vi "ADIS16448 Loop.vi"(8 "error in":errorcluster) -> ()   [LabVIEW 2019]
uses:
  Typedef/ADIS16448 Device Reference.ctl
  Typedef/ADIS16448 Hardware Configuration.ctl
  <vilib>/Rock Robotics/WPI/SPI/WPI_SPIMode.ctl
  <vilib>/Rock Robotics/SystemInterfaces/DIO/FPGA_DIOChannel.ctl
  <vilib>/Rock Robotics/SystemInterfaces/spilib/spi_bus.ctl
  Typedef/ADIS16448 Status.ctl
  Typedef/ADIS16448 Data.ctl
  Typedef/ADIS16448 Process.ctl
  Typedef/ADIS16448 Command Type.ctl
  <vilib>/Rock Robotics/SystemInterfaces/CounterEncoderSourceConvertion/FPGA_CounterEncoderSourceConvertionLVSourceType.ctl
  <vilib>/Rock Robotics/SystemInterfaces/DIO/FPGA_DIODigitalSourceChannel.ctl
  <vilib>/Rock Robotics/SystemInterfaces/AnalogTrigger/FPGA_AnalogTriggerIndex.ctl
  <vilib>/Rock Robotics/SystemInterfaces/AnalogTrigger/FPGA_AnalogTriggerOutType.ctl
  <vilib>/Rock Robotics/WPI/SPI/WPI_SPIDevRef.ctl
  Typedef/ADIS16448 Register.ctl
  <vilib>/Rock Robotics/WPI/Counter/WPI_CounterDigitalInputToDigitalSource.vi
  <vilib>/ptbypt/NI_PtbyPt.lvlib
panel:
  in  "Calibration Time":i32
  in  "element":T1
  in  "ADIS16448DevRef":T2={"DevStatus"={"status"=FALSE, "code"=0, "source"=""}, "Hardware Config"={"SPI Clock Rate (Hz)"=1000000.0, "IMU SPI Mode (3)"=enum."Mode 3 (Clk Idle High,Sample on Trailing)", "IMU Reset Pin"=enum."SPI Port CS2", "IMU SPI Bus"=enum."SPI On-Board, CS0", "IMU Data Ready Pin"=enum."SPI Port CS1", "Stall Config"={"Pow2BytesPerRead"=255, "StallTicks"=640, "CsToSclkTicks"=5}, "IMU Status LED Pin"=enum."DIO MXP 9"}, "Calibration Complete"=refnum, "Status FIFO"=refnum, "Last Value Reference"=refnum, "Sychronous Process VI"=refnum, "Cmd FIFO"=refnum, "Source"={"DevStatus"={"status"=FALSE, "code"=0, "source"=""}, "AnalogTriggerMode?"=FALSE, "DigitalMode"={"DIO Channel"=enum."Disabled"}, "AnalogTriggerMode"={"AnalogTriggerIndex"=enum."Trig 0", "OutputType"=enum."InWindow"}}, "Data FIFO"=refnum, "IMU Status LED Pin"=enum."DIO MXP 9", "Calibration Time"=5}
  in  "Main Name":string
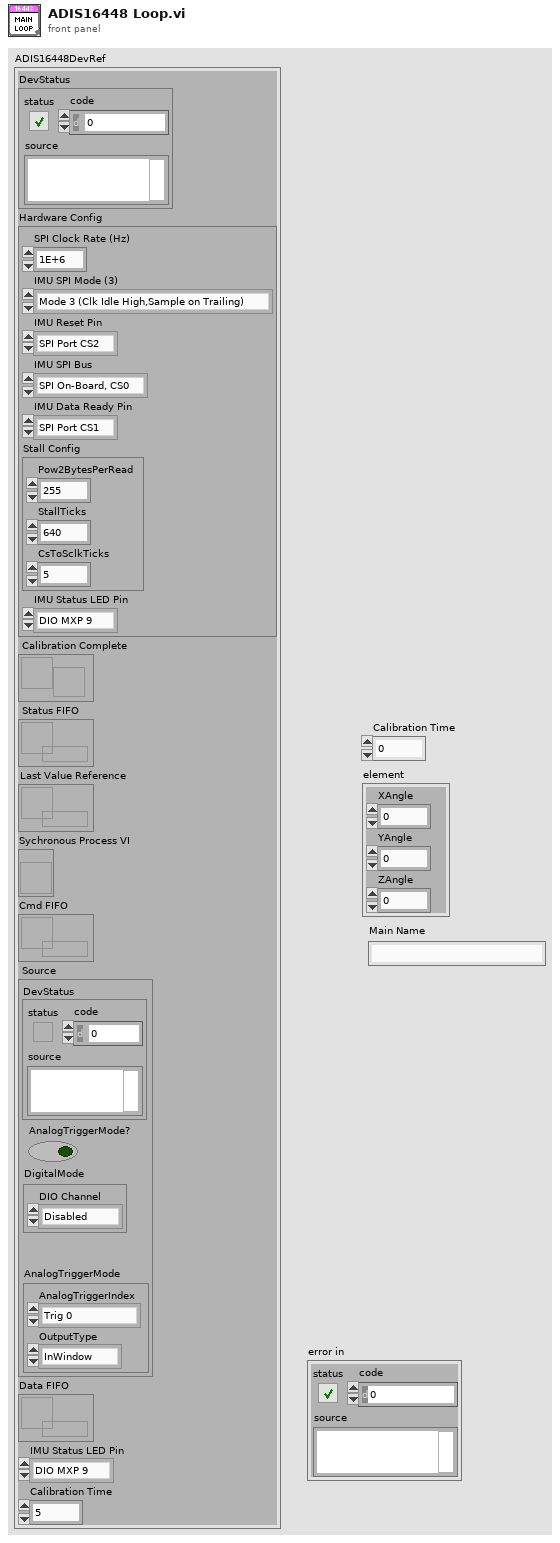
[diagram p1: front panel]
types:
  T1 = typedef "ADIS16448 Data.ctl" = cluster{"XAngle":dbl, "YAngle":dbl, "ZAngle":dbl}
  T2 = typedef "ADIS16448 Device Reference.ctl" = cluster{"DevStatus":errorcluster, "Hardware Config":T3, "Calibration Complete":refnum<notifier>, "Status FIFO":refnum<k33>, "Last Value Reference":refnum<data-value>, "Sychronous Process VI":T7, "Cmd FIFO":refnum<k33>, "Source":T8, "Data FIFO":refnum<k33>, "IMU Status LED Pin":T5, "Calibration Time":u32}
  T3 = typedef "ADIS16448 Hardware Configuration.ctl" = cluster{"SPI Clock Rate (Hz)":dbl, "IMU SPI Mode (3)":T4, "IMU Reset Pin":T5, "IMU SPI Bus":T6, "IMU Data Ready Pin":T5, "Stall Config":cluster{"Pow2BytesPerRead":u8, "StallTicks":u16, "CsToSclkTicks":u8}, "IMU Status LED Pin":T5}
  T4 = typedef "WPI_SPIMode.ctl" = enum16{"Mode 0 (Clk Idle Low,Sample on Leading)", "Mode 1 (Clk Idle Low,Sample on Trailing)", "Mode 2 (Clk Idle High,Sample on Leading)", "Mode 3 (Clk Idle High,Sample on Trailing)"}
  T5 = typedef "FPGA_DIOChannel.ctl" = enum8{"DIO 0", "DIO 1", "DIO 2", "DIO 3", "DIO 4", "DIO 5", "DIO 6", "DIO 7", "DIO 8", "DIO 9", "DIO MXP 0", "DIO MXP 1", "DIO MXP 2", "DIO MXP 3", "DIO MXP 4", "DIO MXP 5", "DIO MXP 6", "DIO MXP 7", "DIO MXP 8", "DIO MXP 9", "DIO MXP 10", "DIO MXP 11", "DIO MXP 12", "DIO MXP 13", "DIO MXP 14", "DIO MXP 15", "SPI Port CS1", "SPI Port CS2", "SPI Port CS3", "SPI Port MISO", "SPI Port MOSI", "Invalid"}
  T6 = typedef "spi_bus.ctl" = enum16{"SPI On-Board, CS0", "SPI On-Board, CS1", "SPI On-Board, CS2", "SPI On-Board, CS3", "SPI MXP", "Invalid"}
  T7 = typedef "ADIS16448 Process.ctl" = refnum<vi>
  T8 = typedef "FPGA_CounterEncoderSourceConvertionLVSourceType.ctl" = cluster{"DevStatus":errorcluster, "AnalogTriggerMode?":bool, "DigitalMode":cluster{"DIO Channel":T9}, "AnalogTriggerMode":cluster{"AnalogTriggerIndex":T10, "OutputType":T11}}
  T9 = typedef "FPGA_DIODigitalSourceChannel.ctl" = enum8{"DIO 0", "DIO 1", "DIO 2", "DIO 3", "DIO 4", "DIO 5", "DIO 6", "DIO 7", "DIO 8", "DIO 9", "DIO MXP 0", "DIO MXP 1", "DIO MXP 2", "DIO MXP 3", "DIO MXP 4", "DIO MXP 5", "DIO MXP 6", "DIO MXP 7", "DIO MXP 8", "DIO MXP 9", "DIO MXP 10", "DIO MXP 11", "DIO MXP 12", "DIO MXP 13", "DIO MXP 14", "DIO MXP 15", "SPI Port CS1", "SPI Port CS2", "SPI Port CS3", "SPI Port MISO", "SPI Port MOSI", "Disabled"}
  T10 = typedef "FPGA_AnalogTriggerIndex.ctl" = enum8{"Trig 0", "Trig 1", "Trig 2", "Trig 3", "Trig 4", "Trig 5", "Trig 6", "Trig 7", "Invalid"}
  T11 = typedef "FPGA_AnalogTriggerOutType.ctl" = enum16{"InWindow", "TriggerState", "Rising", "Falling"}
  T12 = typedef "WPI_SPIDevRef.ctl" = cluster{"DevStatus":errorcluster, "Handle":i32, "SPI Bus":T6}
  T13 = cluster{"SPIDevRef":T12, "Data Counter":u16, "Reset":bool, "Digital Source":T8, "Bytes Per Sample":u32, "Data":dbl[], "ADIS16448DevRef":T2, "TimeStampPrev":u32, "Sensor to Robot Rotation":dbl[][], "AutoSPI Active?":bool, "Offsets":dbl[], "Offset Counter":i32, "Data Header":u8[], "Zero Byte Count":u8, "Running Offset":dbl[]}
  T14 = typedef "ADIS16448 Status.ctl" = cluster{"Calibrated?":bool, "IMU Detected?":bool}
  T15 = typedef "ADIS16448 Register.ctl" = u8
  T16 = typedef "ADIS16448 Command Type.ctl" = cluster{"Command":enum16{"None", "Reset", "Rewrite Config", "Start Recal", "Recalibrate", "Recal Complete", "Exit Auto SPI", "Start Auto SPI", "Configure Cal"}, "Data":u32}
  T17 = typedef "WPI_DigitalOutputDevRef.ctl" = cluster{"DIO Channel":T5, "DevStatus":errorcluster}
  T18 = typedef "WPI_DigitalInputDevRef.ctl" = cluster{"DevStatus":errorcluster, "DIO Channel":T5}
  T19 = cluster{"Pow2BytesPerRead":u8, "StallTicks":u16, "CsToSclkTicks":u8}
  T20 = enum16{"None", "Reset", "Rewrite Config", "Start Recal", "Recalibrate", "Recal Complete", "Exit Auto SPI", "Start Auto SPI", "Configure Cal"}
  T21 = enum32{"Bad", "Idle", "Run top level", "Running"}
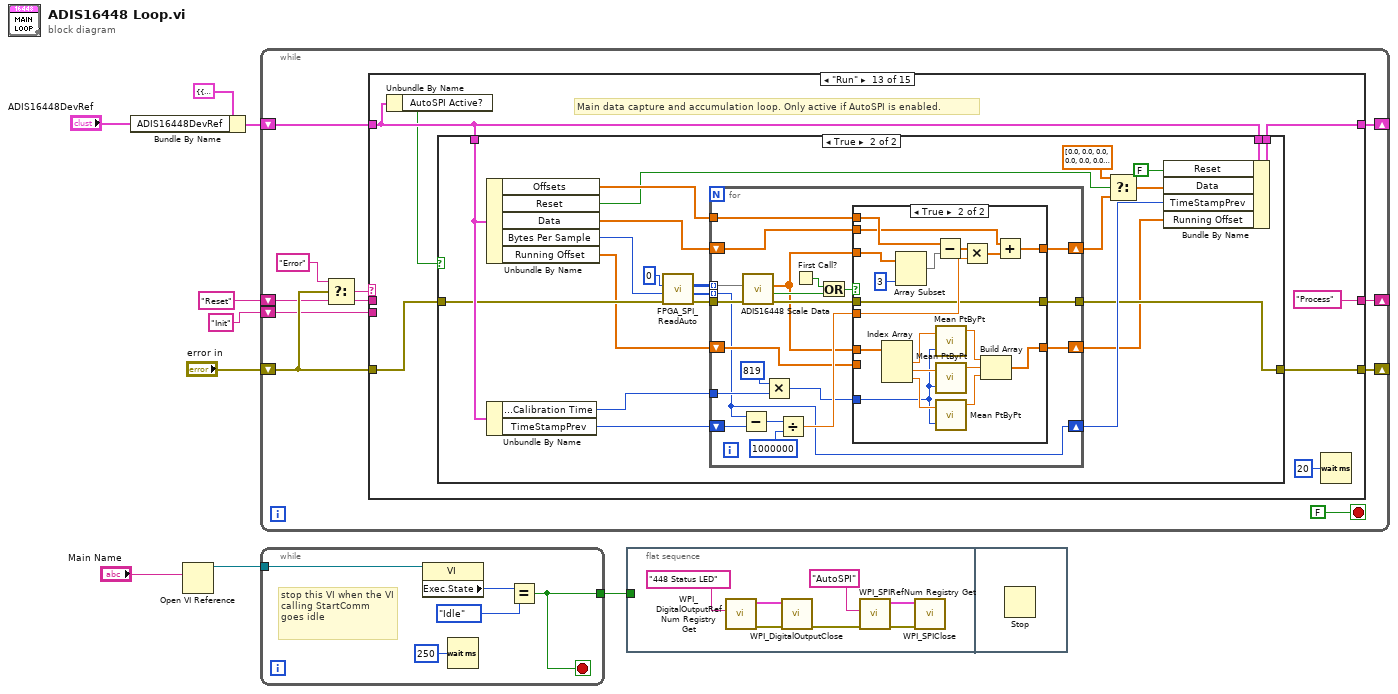
[diagram p0: block diagram]
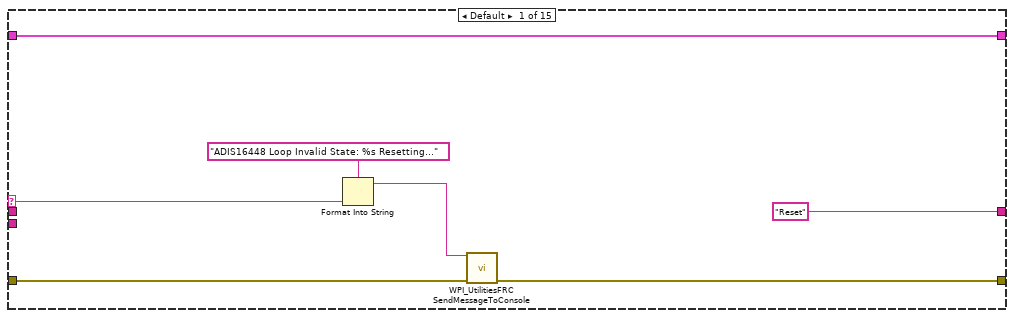
[diagram p2: hidden frame]
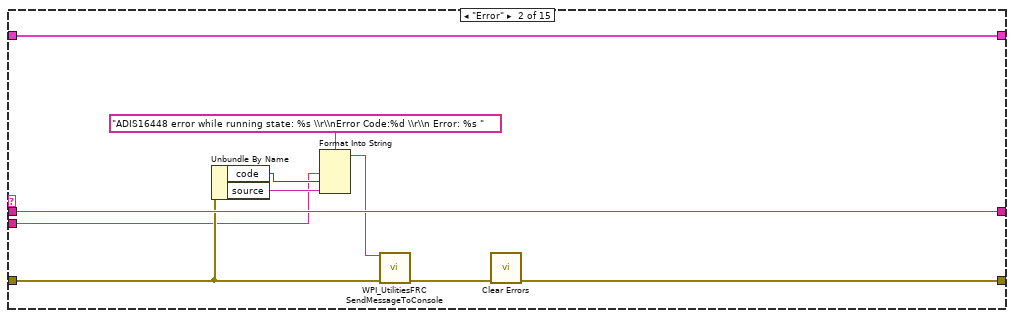
[diagram p3: hidden frame]
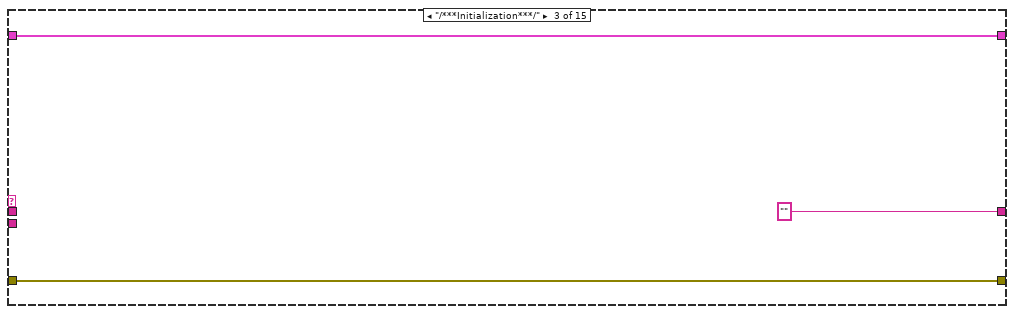
[diagram p4: hidden frame]
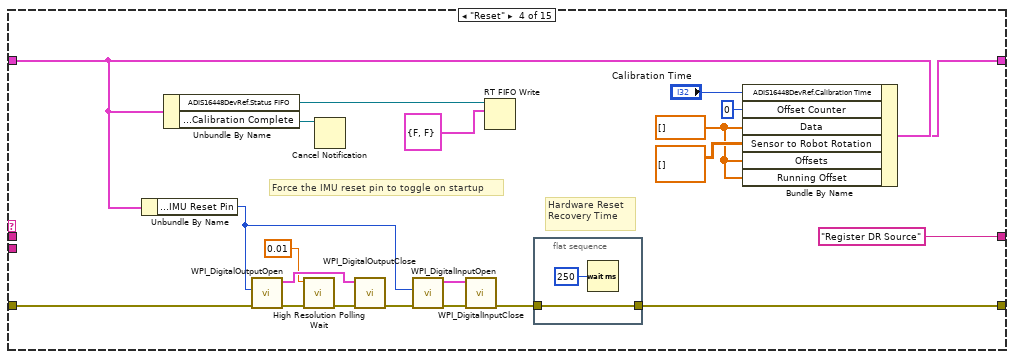
[diagram p5: hidden frame]
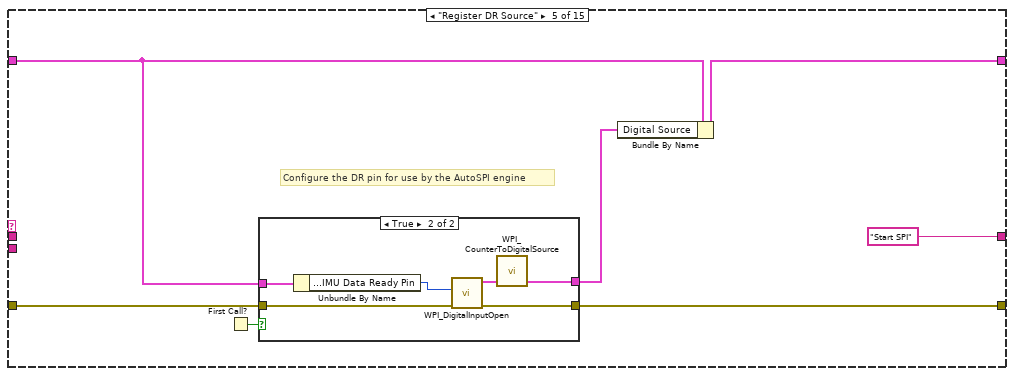
[diagram p6: hidden frame]
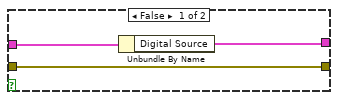
[diagram p7: hidden frame]
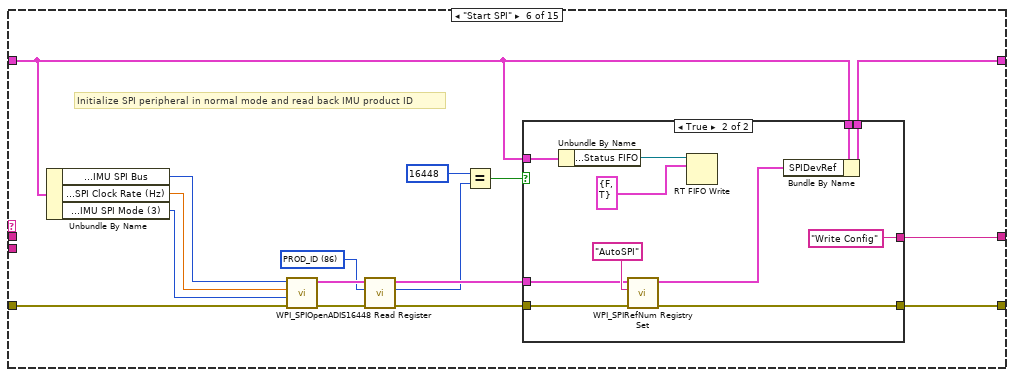
[diagram p8: hidden frame]
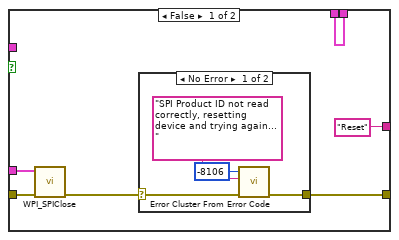
[diagram p9: hidden frame]
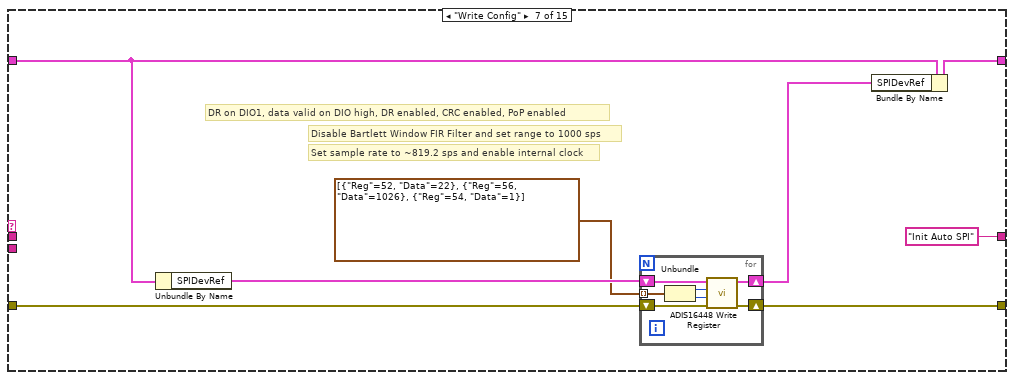
[diagram p11: hidden frame]
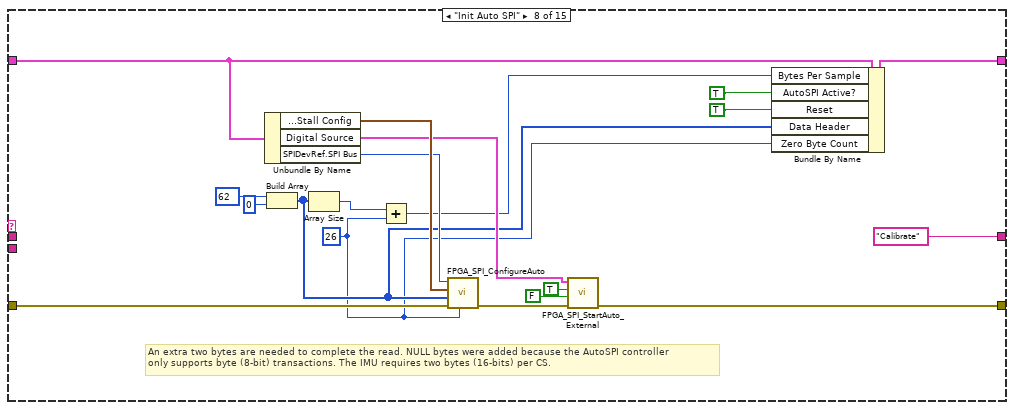
[diagram p12: hidden frame]
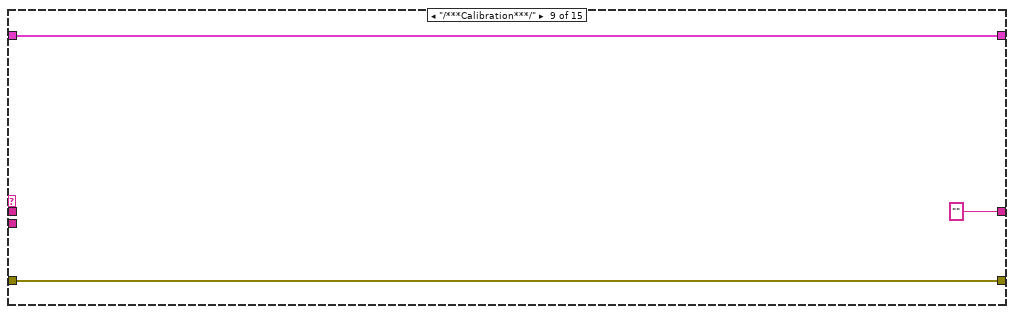
[diagram p13: hidden frame]
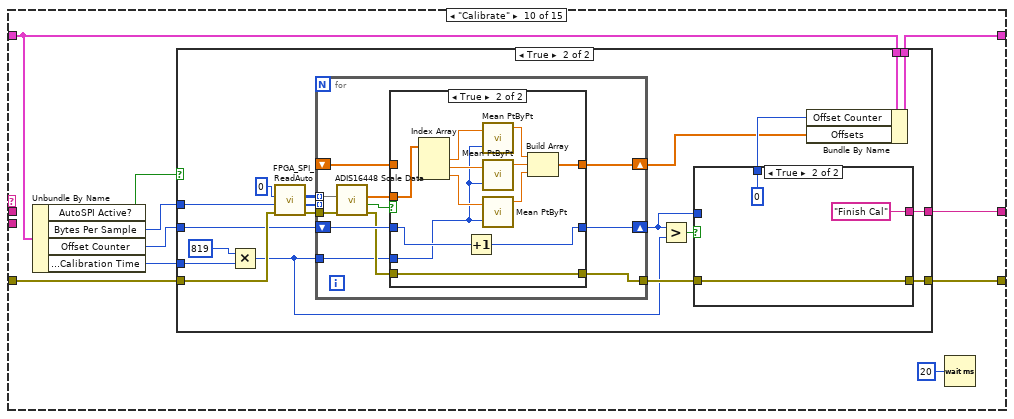
[diagram p14: hidden frame]
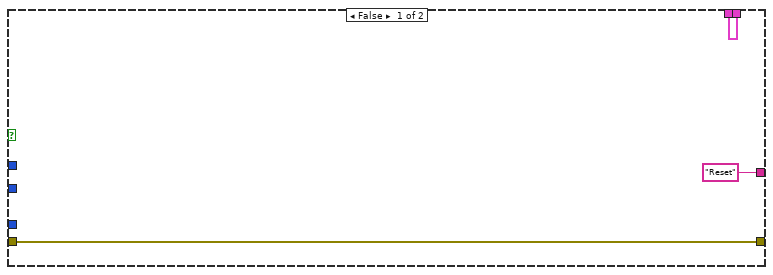
[diagram p15: hidden frame]
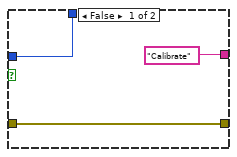
[diagram p16: hidden frame]
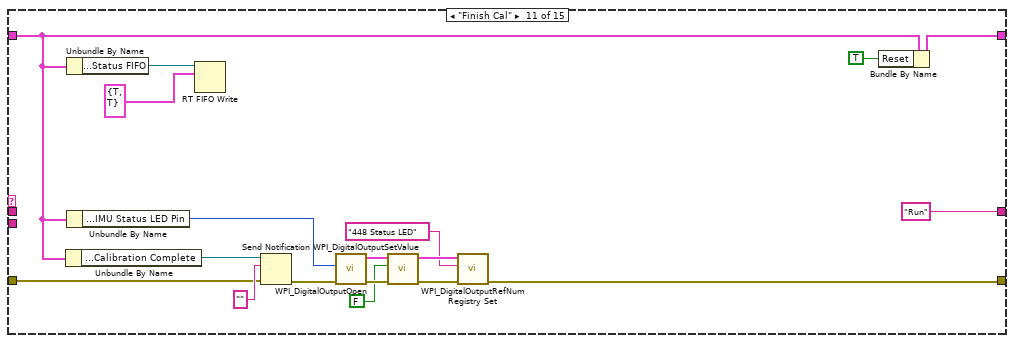
[diagram p18: hidden frame]
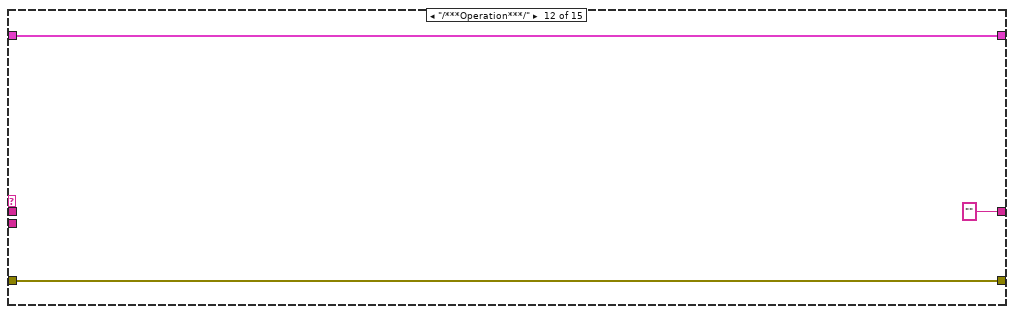
[diagram p19: hidden frame]
diagram:
  n1 = Bundle By Name(cluster=T13 {"SPIDevRef"={"DevStatus"={"status"=FALSE, "code"=0, "source"=""}, "Handle"=0, "SPI Bus"=enum."SPI On-Board, CS0"}, "Data Counter"=0, "Reset"=FALSE, "Digital Source"={"DevStatus"={"status"=FALSE, "code"=0, "source"=""}, "AnalogTriggerMode?"=FALSE, "DigitalMode"={"DIO Channel"=enum."DIO 1"}, "AnalogTriggerMode"={"AnalogTriggerIndex"=enum."Trig 0", "OutputType"=enum."InWindow"}}, "Bytes Per Sample"=0, "Data"=[0.0, 0.0, 0.0, 0.0, 0.0, 0.0, 0.0, 0.0], "ADIS16448DevRef"={"DevStatus"={"status"=FALSE, "code"=0, "source"=""}, "Hardware Config"={"SPI Clock Rate (Hz)"=1000000.0, "IMU SPI Mode (3)"=enum."Mode 3 (Clk Idle High,Sample on Trailing)", "IMU Reset Pin"=enum."SPI Port CS2", "IMU SPI Bus"=enum."SPI On-Board, CS0", "IMU Data Ready Pin"=enum."SPI Port CS1", "Stall Config"={"Pow2BytesPerRead"=255, "StallTicks"=640, "CsToSclkTicks"=5}, "IMU Status LED Pin"=enum."DIO MXP 9"}, "Calibration Complete"=refnum, "Status FIFO"=refnum, "Last Value Reference"=refnum, "Sychronous Process VI"=refnum, "Cmd FIFO"=refnum, "Source"={"DevStatus"={"status"=FALSE, "code"=0, "source"=""}, "AnalogTriggerMode?"=FALSE, "DigitalMode"={"DIO Channel"=enum."Disabled"}, "AnalogTriggerMode"={"AnalogTriggerIndex"=enum."Trig 0", "OutputType"=enum."InWindow"}}, "Data FIFO"=refnum, "IMU Status LED Pin"=enum."DIO MXP 9", "Calibration Time"=5}, "TimeStampPrev"=0, "Sensor to Robot Rotation"=[], "AutoSPI Active?"=TRUE, "Offsets"=[0.0, 0.0, 0.0, 0.0, 0.0, 0.0, 0.0, 0.0], "Offset Counter"=0, "Data Header"=[], "Zero Byte Count"=0, "Running Offset"=[0.0, 0.0, 0.0, 0.0, 0.0, 0.0, 0.0, 0.0]}, "ADIS16448DevRef"="ADIS16448DevRef") -> (w5:T13)
  n2 = Open VI Reference(vi path="Main Name") -> (vi reference=w8:refnum<vi>)  [unwired: 3 in, 3 out]
  n3 = while {
    shift-right: [w15] -> _
    shift-left: "Reset" -> [w12]
    shift-right: [w17] -> _
    shift-left: w5 -> [w18]
    shift-right: [w16] -> _
    shift-left: "error in" -> [w14]
    shift-left: "Init" -> [w10]
    stop <- FALSE stop-if-true
    n4 = Select(t="Error", s=w14, f=w12) -> (s? t:f=w13:string)
    n5 = case shown="\"Run\"" w13 {
      selector: w13 -> [w25 _ _ _ _ _ _ _ _ _ _ _ _ _ _]
      tunnel: w18 -> [w26 w36 w39 w55 w64 w83 w119 w145 w153 w155 w227 w238 w240 w324 w334]
      tunnel: [w26 w36 w39 w54 w68 w88 w118 w144 w153 w160 w234 w238 w244 w324 w340] -> w17
      tunnel: w14 -> [w24 w32 w38 w48 w67 w94 w122 w149 w152 w162 w228 w237 w243 w322 w342]
      tunnel: [w23 w33 w38 w59 w65 w87 w121 w132 w152 w161 w220 w237 w242 w321 w341] -> w16
      tunnel: ["Reset" w35 "" "Register DR Source" "Start SPI" w89 "Init Auto SPI" "Calibrate" "" w156 "Run" "" "Process" "Run Cmds" w332] -> w15
      tunnel: w12 -> [_ w35 _ _ _ _ _ _ _ _ _ _ _ _ _]
      tunnel: w10 -> [_ w27 _ _ _ _ _ _ _ _ _ _ _ _ _]
      frame Default {
        n6 = Format Into String(format string="ADIS16448 Loop Invalid State: %s Resetting...", w25) -> (resulting string=w22:string)  [unwired: 2 in, 1 out]
        n7 = call <vilib>:"WPI_UtilitiesFRC SendMessageToConsole.vi"("Message"=w22, "error in (no error)"=w24) -> ("error out"=w23:errorcluster)  [unwired: 13 in]
      }
      frame "Error" {
        n8 = Unbundle By Name(w32) -> ("code"=w29:i32, "source"=w28:string)
        n9 = Format Into String(format string="ADIS16448 error while running state: %s \\r\\nError Code:%d \\r\\n Error: %s ", w27, w29, w28) -> (resulting string=w31:string)  [unwired: 2 in, 1 out]
        n10 = call <vilib>:"WPI_UtilitiesFRC SendMessageToConsole.vi"("Message"=w31, "error in (no error)"=w32) -> ("error out"=w34:errorcluster)  [unwired: 13 in]
        n11 = call <vilib>:"Clear Errors.vi"("error in (no error)"=w34) -> ("error out"=w33:errorcluster)  [unwired: 5 in, 1 out]
      }
      frame "/***Initialization***/" {
      }
      frame "Reset" {
        w40 = dbl[] [] ("Data")
        # "Hardware Reset Recovery Time"
        # "Force the IMU reset pin to toggle on startup"
        n12 = Unbundle By Name(w55) -> ("ADIS16448DevRef.Hardware Config.IMU Reset Pin"=w44:T5)
        n13 = Unbundle By Name(w55) -> ("ADIS16448DevRef.Status FIFO"=w57:refnum<k33>, "ADIS16448DevRef.Calibration Complete"=w58:refnum<notifier>)
        n14 = call <vilib>:"WPI_DigitalOutputOpen.vi"("error in (no error)"=w48, "DIO Channel"=w44) -> ("error out"=w46:errorcluster, "DigitalOutputDevRef"=w53:T17)  [unwired: 8 in]
        n15 = call <vilib>:"High Resolution Polling Wait.vi"("error in (no error)"=w46, "seconds to wait"=0.01) -> ("error out"=w47:errorcluster)  [unwired: 9 in]
        n16 = Cancel Notification(0:w58) -> ()  [unwired: 1 in, 3 out]
        n17 = call <vilib>:"WPI_DigitalOutputClose.vi"("error in (no error)"=w47, "DigitalOutputDevRef"=w53) -> ("error out"=w50:errorcluster)  [unwired: 9 in]
        n18 = call <vilib>:"WPI_DigitalInputOpen.vi"("error in (no error)"=w50, "DIO Channel"=w44) -> ("error out"=w51:errorcluster, "DigitalInputDevRef"=w52:T18)  [unwired: 8 in]
        n19 = call <vilib>:"WPI_DigitalInputClose.vi"("error in (no error)"=w51, "DigitalInputDevRef"=w52) -> ("error out"=w49:errorcluster)  [unwired: 9 in]
        n20 = RT FIFO Write(0:w57, 1:T14 {"Calibrated?"=FALSE, "IMU Detected?"=FALSE} ("element")) -> ()  [unwired: 3 in, 4 out]
        n21 = flat-sequence {
          tunnel: [w62] -> w59
          tunnel: w49 -> [w62]
          frame #0 {
            n22 = Wait (ms)(milliseconds to wait=u32 250) -> ()  [unwired: 1 out]
          }
        }
        n23 = Bundle By Name(cluster=w55, "ADIS16448DevRef.Calibration Time"="Calibration Time", "Offset Counter"=0, "Data"=w40, "Sensor to Robot Rotation"=dbl[][] [], "Offsets"=w40, "Running Offset"=w40) -> (w54:T13)
      }
      frame "Register DR Source" {
        # "Configure the DR pin for use by the AutoSPI engine"
        n24 = First Call?() -> (First Call?: T/F=w63:bool)
        n25 = case shown="True" w63 {
          tunnel: w67 -> [w70 w78]
          tunnel: w64 -> [w72 w76]
          tunnel: [w71 w74] -> w66
          tunnel: [w70 w73] -> w65
          frame False {
            n26 = Unbundle By Name(w72) -> ("Digital Source"=w71:T8)
          }
          frame True {
            n27 = Unbundle By Name(w76) -> ("ADIS16448DevRef.Hardware Config.IMU Data Ready Pin"=w75:T5)
            n28 = call <vilib>:"WPI_DigitalInputOpen.vi"("error in (no error)"=w78, "DIO Channel"=w75) -> ("error out"=w73:errorcluster, "DigitalInputDevRef"=w77:T18)  [unwired: 8 in]
            n29 = call-poly <vilib>:"WPI_CounterToDigitalSource.vi"("DigitalInputDevRef"=w77) -> ("Digital Source"=w74:T8)  [unwired: 6 in]
          }
        }
        n30 = Bundle By Name(cluster=w64, "Digital Source"=w66) -> (w68:T13)
      }
      frame "Start SPI" {
        w82 = T15 86 items=["FLASH_CNT"=0, "Reserved 1"=2, "XGYRO_OUT"=4, "YGYRO_OUT"=6, "ZGYRO_OUT"=8, "XACCL_OUT"=10, "YACCL_OUT"=12, "ZACCL_OUT"=14, "XMAGN_OUT"=16, "YMAGN_OUT"=18, "ZMAGN_OUT"=20, "BARO_OUT"=22, "TEMP_OUT"=24, "XGYRO_OFF"=26, "YGYRO_OFF"=28, "ZGYRO_OFF"=30, "XACCL_OFF"=32, "YACCL_OFF"=34, "ZACCL_OFF"=36, "XMAGN_HIC"=38, "YMAGN_HIC"=40, "ZMAGN_HIC"=42, "XMAGN_SIC"=44, "YMAGN_SIC"=46, "ZMAGN_SIC"=48, "GPIO_CTRL"=50, "MSC_CTRL"=52, "SMPL_PRD"=54, "SENS_AVG"=56, "SEQ_CNT"=58, "DIAG_STAT"=60, "GLOB_CMD"=62, "ALM_MAG1"=64, "ALM_MAG2"=66, "ALM_SMPL1"=68, "ALM_SMPL2"=70, "ALM_CTRL"=72, "Reserved 2"=74, "Reserved 3"=76, "Reserved 4"=78, "Reserved 5"=80, "LOT_ID1"=82, "LOT_ID2"=84, "PROD_ID"=86, "SERIAL_NUM"=88] ("ADIS16448 Register")
        # "Initialize SPI peripheral in normal mode and read back IMU product ID"
        n31 = Unbundle By Name(w83) -> ("ADIS16448DevRef.Hardware Config.IMU SPI Bus"=w90:T6, "ADIS16448DevRef.Hardware Config.SPI Clock Rate (Hz)"=w91:dbl, "ADIS16448DevRef.Hardware Config.IMU SPI Mode (3)"=w92:T4)
        n32 = call <vilib>:"WPI_SPIOpen.vi"("error in"=w94, "Mode (3)"=w92, "Clock Rate (Hz)"=w91, "SPI Bus"=w90) -> ("error out"=w86:errorcluster, "SPIDevRef"=w85:T12)  [unwired: 6 in]
        n33 = call "ADIS16448 Read Register.vi"("error in (no error)"=w86, "ADIS16448 Register"=w82, "SPIDevRef in"=w85) -> ("error out"=w80:errorcluster, "Register Value"=w79:u16, "SPIDevRef out"=w81:T12)  [unwired: 6 in]
        n34 = Equal?(x=u16 16448 ("y"), y=w79) -> (x = y?=w93:bool)
        n35 = case shown="True" w93 {
          tunnel: ["Reset" "Write Config"] -> w89
          tunnel: w83 -> [w99 w115]
          tunnel: [w99 w114] -> w88
          tunnel: [w98 w109] -> w87
          tunnel: w80 -> [w97 w110]
          tunnel: w81 -> [w96 w111]
          tunnel: w83 -> [_ w106]
          frame False {
            n36 = call <vilib>:"WPI_SPIClose.vi"("error in (no error)"=w97, "SPIDevRef"=w96) -> ("error out"=w95:errorcluster)  [unwired: 9 in]
            n37 = case shown="No Error" w95 {
              selector: w95 -> [w103 w105]
              tunnel: [w104 w105] -> w98
              frame No Error {
                n38 = call <vilib>:"Error Cluster From Error Code.vi"("error in (no error)"=w103, "error message (\"\")"="SPI Product ID not read correctly, resetting device and trying again..." ("error message (\"\")"), "error code (0)"=-8106) -> ("error out"=w104:errorcluster)  [unwired: 6 in]
              }
              frame Error {
              }
            }
          }
          frame True {
            n39 = Unbundle By Name(w106) -> ("ADIS16448DevRef.Status FIFO"=w108:refnum<k33>)
            n40 = call <vilib>:"WPI_SPIRefNum Registry Set.vi"("error in (no error)"=w110, "refnum name"="AutoSPI", "SPIDevRef"=w111) -> ("error out"=w109:errorcluster, "SPIDevRef"=w113:T12)  [unwired: 7 in]
            n41 = RT FIFO Write(0:w108, 1:T14 {"Calibrated?"=FALSE, "IMU Detected?"=TRUE} ("element")) -> ()  [unwired: 3 in, 4 out]
            n42 = Bundle By Name(cluster=w115, "SPIDevRef"=w113) -> (w114:T13)
          }
        }
      }
      frame "Write Config" {
        # "DR on DIO1, data valid on DIO high, DR enabled, CRC enabled, PoP enabled"
        # "Set sample rate to ~819.2 sps and enable internal clock"
        # "Disable Bartlett Window FIR Filter and set range to 1000 sps"
        n43 = Unbundle By Name(w119) -> ("SPIDevRef"=w123:T12)
        n44 = for {
          tunnel: cluster{"Reg":T15, "Data":u16}[] [{"Reg"=52, "Data"=22}, {"Reg"=56, "Data"=1026}, {"Reg"=54, "Data"=1}] -> [w131] mode=indexing
          shift-right: [w127] -> w121
          shift-left: w122 -> [w126]
          shift-right: [w125] -> w117
          shift-left: w123 -> [w128]
          n45 = Unbundle(w131) -> ("Reg"=w130:T15, "Data"=w129:u16)
          n46 = call "ADIS16448 Write Register.vi"("error in (no error)"=w126, "Data"=w129, "Register"=w130, "SPIDevRef in"=w128) -> ("error out"=w127:errorcluster, "SPIDevRef out"=w125:T12)  [unwired: 6 in]
        }
        n47 = Bundle By Name(cluster=w119, "SPIDevRef"=w117) -> (w118:T13)
      }
      frame "Init Auto SPI" {
        w133 = u8 26 ("dimension size")
        # "An extra two bytes are needed to complete the read. NULL bytes were added because the AutoSPI controller \nonly supports byte (8-bit) transactions. The IMU requires two bytes (16-bits) per CS."
        n48 = Unbundle By Name(w145) -> ("ADIS16448DevRef.Hardware Config.Stall Config"=w143:T19, "Digital Source"=w141:T8, "SPIDevRef.SPI Bus"=w140:T6)
        n49 = Build Array(u8 62 ("hi"), u8 0 ("element")) -> (w134:u8[])
        n50 = Array Size(array=w134) -> (size(s)=w138:i32)
        n51 = Add(x=w138, y=w133) -> (x+y=w135:i32)
        n52 = call <vilib>:"FPGA_SPI_ConfigureAuto.vi"("SPI Auto Zero Byte Count"=w133, "error in"=w149, "SPI Auto TX Byte Array"=w134, "Stall Config"=w143, "SPI Bus"=w140) -> ("error out"=w148:errorcluster)  [unwired: 6 in]
        n53 = call <vilib>:"FPGA_SPI_StartAuto_External.vi"("error in (no error)"=w148, "Falling Edge"=FALSE, "Rising Edge"=TRUE, "Source"=w141) -> ("error out"=w132:errorcluster)  [unwired: 7 in]
        n54 = Bundle By Name(cluster=w145, "Bytes Per Sample"=w135, "AutoSPI Active?"=TRUE, "Reset"=TRUE, "Data Header"=w134, "Zero Byte Count"=w133) -> (w144:T13)
      }
      frame "/***Calibration***/" {
      }
      frame "Calibrate" {
        n55 = Unbundle By Name(w155) -> ("AutoSPI Active?"=w163:bool, "Bytes Per Sample"=w159:u32, "Offset Counter"=w158:i32, "ADIS16448DevRef.Calibration Time"=w157:u32)
        n56 = case shown="True" w163 {
          tunnel: [w166 w185] -> w160
          tunnel: w162 -> [w165 w180]
          tunnel: [w165 w170] -> w161
          tunnel: w155 -> [w166 w181]
          tunnel: w159 -> [_ w178]
          tunnel: w158 -> [_ w175]
          tunnel: w157 -> [_ w176]
          tunnel: ["Reset" w171] -> w156
          frame False {
          }
          frame True {
            n57 = Multiply(x=819, y=w176) -> (x*y=w167:u32)
            n58 = call <vilib>:"FPGA_SPI_ReadAuto.vi"("error in (no error)"=w180, "Bytes per Sample"=w178, "Samples to Read"=u32 0) -> ("error out"=w179:errorcluster, "Timestamps"=w182:u32[], "Data"=w183:u8[][])  [unwired: 6 in]
            n59 = for {
              tunnel: w183 -> [w202] mode=indexing
              tunnel: w182 -> [_] mode=indexing
              tunnel: w179 -> [w201]
              tunnel: [w196] -> w169
              shift-right: [w197] -> w173
              shift-left: w175 -> [w198]
              shift-right: [w194] -> w168
              shift-left: _ -> [w193]
              tunnel: w167 -> [w192]
              n60 = call "ADIS16448 Scale Data.vi"("error in (no error)"=w201, "New Data In"=w202) -> ("error out"=w195:errorcluster, "Data Good?"=w200:bool, "Data Out"=w199:dbl[])  [unwired: 7 in]
              n61 = case shown="True" w200 {
                tunnel: w199 -> [_ w211]
                tunnel: w198 -> [w205 w208]
                tunnel: [w205 w207] -> w197
                tunnel: [w204 w209] -> w196
                tunnel: w195 -> [w204 w209]
                tunnel: [w203 w210] -> w194
                tunnel: w193 -> [w203 _]
                tunnel: w192 -> [_ w206]
                frame False {
                }
                frame True {
                  n62 = Index Array(array=w211) -> (element #1=w212:dbl, element #2=w213:dbl, element #3=w214:dbl)  [unwired: 3 in]
                  n63 = Increment(x=w208) -> (x+1=w207:i32)
                  n64 = call <vilib>:"Mean PtByPt.vi"("x"=w212, "sample length"=w206) -> ("mean"=w215:dbl)  [unwired: 2 in, 1 out]
                  n65 = call <vilib>:"Mean PtByPt.vi"("x"=w213, "sample length"=w206) -> ("mean"=w216:dbl)  [unwired: 2 in, 1 out]
                  n66 = call <vilib>:"Mean PtByPt.vi"("x"=w214, "sample length"=w206) -> ("mean"=w217:dbl)  [unwired: 2 in, 1 out]
                  n67 = Build Array(w215, w216, w217) -> (w210:dbl[])
                }
              }
            }
            n68 = Greater?(x=w173, y=w167) -> (0:w174:bool)
            n69 = case shown="True" w174 {
              tunnel: w173 -> [w188 _]
              tunnel: [w188 u32 0 ("Offset Counter")] -> w172
              tunnel: ["Calibrate" "Finish Cal"] -> w171
              tunnel: [w186 w189] -> w170
              tunnel: w169 -> [w186 w189]
              frame False {
              }
              frame True {
              }
            }
            n70 = Bundle By Name(cluster=w181, "Offset Counter"=w172, "Offsets"=w168) -> (w185:T13)
          }
        }
        n71 = Wait (ms)(milliseconds to wait=u32 20) -> ()  [unwired: 1 out]
      }
      frame "Finish Cal" {
        n72 = Unbundle By Name(w227) -> ("ADIS16448DevRef.Calibration Complete"=w232:refnum<notifier>)
        n73 = Unbundle By Name(w227) -> ("ADIS16448DevRef.Status FIFO"=w230:refnum<k33>)
        n74 = Unbundle By Name(w227) -> ("ADIS16448DevRef.Hardware Config.IMU Status LED Pin"=w218:T5)
        n75 = RT FIFO Write(0:w230, 1:T14 {"Calibrated?"=TRUE, "IMU Detected?"=TRUE} ("element")) -> ()  [unwired: 3 in, 4 out]
        n76 = Send Notification(notification="", notifier=w232, error in (no error)=w228) -> (error out=w221:errorcluster)  [unwired: 1 out]
        n77 = call <vilib>:"WPI_DigitalOutputOpen.vi"("error in (no error)"=w221, "DIO Channel"=w218) -> ("error out"=w226:errorcluster, "DigitalOutputDevRef"=w225:T17)  [unwired: 8 in]
        n78 = call <vilib>:"WPI_DigitalOutputSetValue.vi"("error in (no error)"=w226, "Value"=FALSE, "DigitalOutputDevRef"=w225) -> ("error out"=w224:errorcluster, "DigitalOutputDevRef"=w223:T17)  [unwired: 7 in]
        n79 = call <vilib>:"WPI_DigitalOutputRefNum Registry Set.vi"("error in (no error)"=w224, "refnum name"="448 Status LED", "DigitalOutputDevRef"=w223) -> ("error out"=w220:errorcluster)  [unwired: 7 in, 1 out]
        n80 = Bundle By Name(cluster=w227, "Reset"=TRUE ("First Run")) -> (w234:T13)
      }
      frame "/***Operation***/" {
      }
      frame "Run" {
        # "Main data capture and accumulation loop. Only active if AutoSPI is enabled."
        n81 = Unbundle By Name(w240) -> ("AutoSPI Active?"=w239:bool)
        n82 = case shown="True" w239 {
          tunnel: [w247 w269] -> w244
          tunnel: w243 -> [w246 w255]
          tunnel: [w246 w252] -> w242
          tunnel: w240 -> [w247 w259]
          tunnel: w240 -> [_ w256]
          frame False {
          }
          frame True {
            n83 = Unbundle By Name(w256) -> ("Offsets"=w253:dbl[], "Reset"=w251:bool, "Data"=w263:dbl[], "Bytes Per Sample"=w267:u32, "Running Offset"=w249:dbl[])
            n84 = Unbundle By Name(w256) -> ("ADIS16448DevRef.Calibration Time"=w250:u32, "TimeStampPrev"=w258:u32)
            n85 = call <vilib>:"FPGA_SPI_ReadAuto.vi"("error in (no error)"=w255, "Bytes per Sample"=w267, "Samples to Read"=u32 0) -> ("error out"=w254:errorcluster, "Timestamps"=w264:u32[], "Data"=w265:u8[][])  [unwired: 6 in]
            n86 = for {
              tunnel: w265 -> [w289] mode=indexing
              tunnel: w264 -> [w270] mode=indexing
              shift-right: [w283] -> w262
              shift-left: w263 -> [w282]
              shift-right: [w270] -> w257
              shift-left: w258 -> [w290]
              tunnel: w254 -> [w288]
              tunnel: w253 -> [w287]
              tunnel: [w280] -> w252
              tunnel: w250 -> [w275]
              shift-right: [w271] -> w248
              shift-left: w249 -> [w272]
              n87 = Subtract(x=w270, y=w290) -> (x-y=w286:u32)
              n88 = call "ADIS16448 Scale Data.vi"("error in (no error)"=w288, "New Data In"=w289) -> ("error out"=w281:errorcluster, "Data Good?"=w278:bool, "Data Out"=w276:dbl[])  [unwired: 7 in]
              n89 = Multiply(x=819, y=w275) -> (x*y=w273:u32)
              n90 = Divide(x=w286, y=u32 1000000) -> (x/y=w284:dbl)
              n91 = First Call?() -> (First Call?: T/F=w277:bool)
              n92 = Or(x=w277, y=w278) -> (x .or. y?=w279:bool)
              n93 = case shown="True" w279 {
                tunnel: w276 -> [_ w311]
                tunnel: w287 -> [_ w309]
                tunnel: w284 -> [_ w307]
                tunnel: [w293 w306] -> w283
                tunnel: w282 -> [w293 w304]
                tunnel: w281 -> [w292 w303]
                tunnel: [w292 w303] -> w280
                tunnel: w276 -> [_ w296]
                tunnel: w273 -> [_ w295]
                tunnel: w272 -> [w291 _]
                tunnel: [w291 w294] -> w271
                frame False {
                }
                frame True {
                  n94 = Index Array(array=w296) -> (element #1=w297:dbl, element #2=w298:dbl, element #3=w299:dbl)  [unwired: 3 in]
                  n95 = Array Subset(array=w311, length=3) -> (w310:dbl[])  [unwired: 1 in]
                  n96 = Subtract(x=w309, y=w310) -> (x-y=w308:dbl[])
                  n97 = call <vilib>:"Mean PtByPt.vi"("x"=w297, "sample length"=w295) -> ("mean"=w300:dbl)  [unwired: 2 in, 1 out]
                  n98 = call <vilib>:"Mean PtByPt.vi"("x"=w298, "sample length"=w295) -> ("mean"=w301:dbl)  [unwired: 2 in, 1 out]
                  n99 = call <vilib>:"Mean PtByPt.vi"("x"=w299, "sample length"=w295) -> ("mean"=w302:dbl)  [unwired: 2 in, 1 out]
                  n100 = Multiply(x=w308, y=w307) -> (x*y=w305:dbl[])
                  n101 = Build Array(w300, w301, w302) -> (w294:dbl[])
                  n102 = Add(x=w304, y=w305) -> (x+y=w306:dbl[])
                }
              }
            }
            n103 = Select(t=dbl[] [0.0, 0.0, 0.0, 0.0, 0.0, 0.0, 0.0, 0.0] ("Angle and Vel"), s=w251, f=w262) -> (s? t:f=w260:dbl[])
            n104 = Bundle By Name(cluster=w259, "Reset"=FALSE ("First Run"), "Data"=w260, "TimeStampPrev"=w257, "Running Offset"=w248) -> (w269:T13)
          }
        }
        n105 = Wait (ms)(milliseconds to wait=u32 20) -> ()  [unwired: 1 out]
      }
      frame "Process" {
        n106 = Unbundle By Name(w324) -> ("ADIS16448DevRef.Sychronous Process VI"=w319:T7, "ADIS16448DevRef.Data FIFO"=w323:refnum<k33>, "Data"=w318:dbl[])
        n107 = Index Array(array=w318) -> (element #1=w317:dbl, element #2=w316:dbl, element #3=w315:dbl)  [unwired: 3 in]
        n108 = Bundle By Name(cluster="element", "XAngle"=w317, "YAngle"=w316, "ZAngle"=w315) -> (w313:T1)
        n109 = RT FIFO Write(0:w323, 1:w313) -> ()  [unwired: 3 in, 4 out]
        n110 = Not A Number/Path/Refnum?(number/path/refnum=w319) -> (NaN/Path/Refnum?=w320:bool)
        n111 = case shown="False" w320 {
          tunnel: w322 -> [w326 w331]
          tunnel: w313 -> [_ _]
          tunnel: [w330 w331] -> w321
          tunnel: w319 -> [w329 _]
          frame False {
            n112 = call-by-ref "?"(reference=w329, error in=w326, 8:"error in (no error)"=w326) -> (error out=w327:errorcluster, 0:"error out"=w328:errorcluster)  [unwired: 10 in, 1 out]
            n113 = Merge Errors(w327, w328) -> (w330:errorcluster)
          }
          frame True {
          }
        }
      }
      frame "Run Cmds" {
        n114 = Unbundle By Name(w334) -> ("ADIS16448DevRef.Cmd FIFO"=w343:refnum<k33>)
        n115 = Unbundle By Name(w334) -> ("ADIS16448DevRef.Status FIFO"=w338:refnum<k33>, "ADIS16448DevRef.Calibration Complete"=w339:refnum<notifier>)
        n116 = RT FIFO Read(0:w343, 1:T16 {"Command"=enum."None", "Data"=0} ("element")) -> (8:w337:refnum<k33>, 9:w336:T16)  [unwired: 2 in, 3 out]
        n117 = Unbundle(w336) -> ("Command"=w333:T20, "Data"=w335:u32)
        n118 = case shown="\"Exit Auto SPI\"" w333 {
          tunnel: w334 -> [w346 w352 w361 w372 w381 w399 w445 w462 w469]
          tunnel: w342 -> [w347 w351 w359 w369 w386 w415 w455 w465 w470]
          tunnel: [w347 w351 w358 w369 w386 w402 w446 w465 w470] -> w341
          tunnel: [w346 w350 w361 w373 w380 w398 w445 w462 w468] -> w340
          tunnel: w339 -> [_ _ _ _ w385 _ _ _ _]
          tunnel: w338 -> [_ _ _ _ w383 w390 _ w463 _]
          tunnel: w337 -> [_ _ w356 w376 _ w413 w457 w459 _]
          tunnel: w335 -> [_ _ _ _ _ _ _ _ w466]
          tunnel: w334 -> [_ _ w355 w374 _ w396 w444 _ _]
          tunnel: ["Run" "Run" "Run" "Run" "Run" w387 "Run" "Run" "Run"] -> w332
          frame "None", Default {
          }
          frame "Reset" {
            n119 = Bundle By Name(cluster=w352, "Reset"=TRUE ("First Run")) -> (w350:T13)
          }
          frame "Rewrite Config" {
            n120 = Unbundle By Name(w355) -> ("SPIDevRef"=w354:T12)
            n121 = RT FIFO Write(0:w356, 1:T16 {"Command"=enum."Start Auto SPI", "Data"=0} ("element")) -> ()  [unwired: 3 in, 4 out]
            n122 = for {
              tunnel: cluster{"Reg":T15, "Data":u16}[] [{"Reg"=52, "Data"=22}, {"Reg"=56, "Data"=1026}, {"Reg"=54, "Data"=1}] -> [w368] mode=indexing
              shift-right: [w364] -> w358
              shift-left: w359 -> [w363]
              shift-right: [w362] -> _
              shift-left: w354 -> [w365]
              n123 = Unbundle(w368) -> ("Reg"=w367:T15, "Data"=w366:u16)
              n124 = call "ADIS16448 Write Register.vi"("error in (no error)"=w363, "Data"=w366, "Register"=w367, "SPIDevRef in"=w365) -> ("error out"=w364:errorcluster, "SPIDevRef out"=w362:T12)  [unwired: 6 in]
            }
          }
          frame "Recalibrate" {
            n125 = Unbundle By Name(w374) -> ("Running Offset"=w371:dbl[])
            n126 = RT FIFO Write(0:w376, 1:T16 {"Command"=enum."Recal Complete", "Data"=0} ("element")) -> ()  [unwired: 3 in, 4 out]
            n127 = Bundle By Name(cluster=w372, "Offsets"=w371) -> (w373:T13)
          }
          frame "Recal Complete" {
            n128 = Send Notification(notification="", notifier=w385) -> ()  [unwired: 1 in, 2 out]
            n129 = RT FIFO Write(0:w383, 1:T14 {"Calibrated?"=TRUE, "IMU Detected?"=TRUE} ("element")) -> ()  [unwired: 3 in, 4 out]
            n130 = Bundle By Name(cluster=w381, "AutoSPI Active?"=TRUE, "Reset"=TRUE) -> (w380:T13)
          }
          frame "Exit Auto SPI" {
            w409 = T15 114 items=["Reserved1"=0, "DIAG_STAT"=2, "X_GYRO_LOW"=4, "X_GYRO_OUT"=6, "Y_GYRO_LOW"=8, "Y_GYRO_OUT"=10, "Z_GYRO_LOW"=12, "Z_GYRO_OUT"=14, "X_ACCL_LOW"=16, "X_ACCL_OUT"=18, "Y_ACCL_LOW"=20, "Y_ACCL_OUT"=22, "Z_ACCL_LOW"=24, "Z_ACCL_OUT"=26, "TEMP_OUT"=28, "TIME_STAMP"=30, "Reseved2"=32, "DATA_CNTR"=34, "X_DELTANG_LOW"=36, "X_DELTANG_OUT"=38, "Y_DELTANG_LOW"=40, "Y_DELTANG_OUT"=42, "Z_DELTANG_LOW"=44, "Z_DELTANG_OUT"=46, "X_DELTVEL_LOW"=48, "X_DELTVEL_OUT"=50, "Y_DELTVEL_LOW"=52, "Y_DELTVEL_OUT"=54, "Z_DELTVEL_LOW"=56, "Z_DELTVEL_OUT"=58, "Reserved3"=60, "Reserved4"=62, "XG_BIAS_LOW"=64, "XG_BIAS_HIGH"=66, "YG_BIAS_LOW"=68, "YG_BIAS_OUT"=70, "ZG_BIAS_LOW"=72, "ZG_BIAS_OUT"=74, "XA_BIAS_LOW"=76, "XA_BIAS_HIGH"=78, "YA_BIAS_LOW"=80, "YA_BIAS_OUT"=82, "ZA_BIAS_LOW"=84, "ZA_BIAS_OUT"=86, "Reserved5"=88, "Reserved6"=90, "FILT_CTRL"=92, "Reserved5"=94, "MSC_CTRL"=96, "UP_SCALE"=98, "DEC_RATE"=100, "NULL_CNFG"=102, "GLOB_CMD"=104, "Reserved6"=106, "FIRM_REV"=108, "FIRM_DM"=110, "FIRM_Y"=112, "PROD_ID"=114, "SERIAL_NUM"=116, "USER_SCR1"=118, "USER_SCR2"=120, "USER_SCR3"=122, "FLSHCNT_LOW"=124, "FLSHCNT_HIGH"=126] ("ADIS16448 Register")
            n131 = Unbundle By Name(w396) -> ("ADIS16448DevRef.Hardware Config.IMU SPI Bus"=w412:T6, "ADIS16448DevRef.Hardware Config.SPI Clock Rate (Hz)"=w411:dbl, "ADIS16448DevRef.Hardware Config.IMU SPI Mode (3)"=w410:T4, "SPIDevRef"=w391:T12)
            n132 = RT FIFO Write(0:w390, 1:T14 {"Calibrated?"=FALSE, "IMU Detected?"=FALSE} ("element")) -> (8:w388:refnum<k33>)  [unwired: 3 in, 3 out]
            n133 = RT FIFO Write(0:w413, 1:T16 {"Command"=enum."Rewrite Config", "Data"=0} ("element")) -> ()  [unwired: 3 in, 4 out]
            n134 = call <vilib>:"WPI_SPIClose.vi"("error in (no error)"=w415, "SPIDevRef"=w391) -> ("error out"=w400:errorcluster)  [unwired: 9 in]
            n135 = call <vilib>:"WPI_DigitalOutputRefNum Registry Get.vi"("error in (no error)"=w400, "refnum name"="448 Status LED") -> ("error out"=w394:errorcluster, "DigitalOutputDevRef"=w393:T17)  [unwired: 8 in]
            n136 = call <vilib>:"WPI_DigitalOutputSetValue.vi"("error in (no error)"=w394, "Value"=TRUE, "DigitalOutputDevRef"=w393) -> ("error out"=w395:errorcluster)  [unwired: 7 in, 1 out]
            n137 = call <vilib>:"WPI_SPIOpen.vi"("error in"=w395, "Mode (3)"=w410, "Clock Rate (Hz)"=w411, "SPI Bus"=w412) -> ("error out"=w408:errorcluster, "SPIDevRef"=w404:T12)  [unwired: 6 in]
            n138 = call "ADIS16448 Read Register.vi"("error in (no error)"=w408, "ADIS16448 Register"=w409, "SPIDevRef in"=w404) -> ("error out"=w405:errorcluster, "Register Value"=w403:u16, "SPIDevRef out"=w406:T12)  [unwired: 6 in]
            n139 = Equal?(x=u16 16448 ("y"), y=w403) -> (x = y?=w407:bool)
            n140 = case shown="True" w407 {
              tunnel: w406 -> [w418 w435]
              tunnel: w405 -> [w419 w434]
              tunnel: [w421 w433] -> w402
              tunnel: w399 -> [w420 w431]
              tunnel: [w420 w430] -> w398
              tunnel: w388 -> [_ w429]
              tunnel: ["Reset" "Run"] -> w387
              frame False {
                n141 = call <vilib>:"WPI_SPIClose.vi"("error in (no error)"=w419, "SPIDevRef"=w418) -> ("error out"=w417:errorcluster)  [unwired: 9 in]
                n142 = case shown="No Error" w417 {
                  selector: w417 -> [w423 w426]
                  tunnel: [w422 w426] -> w421
                  frame No Error {
                    n143 = call <vilib>:"Error Cluster From Error Code.vi"("error in (no error)"=w423, "error message (\"\")"="SPI port did not reset properly" ("error message (\"\")"), "error code (0)"=-8106) -> ("error out"=w422:errorcluster)  [unwired: 6 in]
                  }
                  frame Error {
                  }
                }
              }
              frame True {
                n144 = call <vilib>:"WPI_SPIRefNum Registry Set.vi"("error in (no error)"=w434, "refnum name"="AutoSPI", "SPIDevRef"=w435) -> ("error out"=w433:errorcluster, "SPIDevRef"=w436:T12)  [unwired: 7 in]
                n145 = RT FIFO Write(0:w429, 1:T14 {"Calibrated?"=FALSE, "IMU Detected?"=TRUE} ("element")) -> ()  [unwired: 3 in, 4 out]
                n146 = Bundle By Name(cluster=w431, "SPIDevRef"=w436, "AutoSPI Active?"=FALSE) -> (w430:T13)
              }
            }
          }
          frame "Start Auto SPI" {
            n147 = Unbundle By Name(w444) -> ("SPIDevRef"=w443:T12, "Digital Source"=w442:T8, "ADIS16448DevRef.Hardware Config.Stall Config"=w441:T19, "Data Header"=w440:u8[], "Zero Byte Count"=w439:u8)
            n148 = Unbundle By Name(w443) -> ("SPI Bus"=w456:T6)
            n149 = RT FIFO Write(0:w457, 1:T16 {"Command"=enum."Recal Complete", "Data"=0} ("element")) -> ()  [unwired: 3 in, 4 out]
            n150 = call <vilib>:"FPGA_SPI_ConfigureAuto.vi"("SPI Auto Zero Byte Count"=w439, "error in"=w455, "SPI Auto TX Byte Array"=w440, "Stall Config"=w441, "SPI Bus"=w456) -> ("error out"=w448:errorcluster)  [unwired: 6 in]
            n151 = call <vilib>:"FPGA_SPI_StartAuto_External.vi"("error in (no error)"=w448, "Falling Edge"=FALSE, "Rising Edge"=TRUE, "Source"=w442) -> ("error out"=w452:errorcluster)  [unwired: 7 in]
            n152 = call <vilib>:"WPI_DigitalOutputRefNum Registry Get.vi"("error in (no error)"=w452, "refnum name"="448 Status LED") -> ("error out"=w451:errorcluster, "DigitalOutputDevRef"=w450:T17)  [unwired: 8 in]
            n153 = call <vilib>:"WPI_DigitalOutputSetValue.vi"("error in (no error)"=w451, "Value"=FALSE, "DigitalOutputDevRef"=w450) -> ("error out"=w446:errorcluster)  [unwired: 7 in, 1 out]
          }
          frame "Start Recal" {
            n154 = RT FIFO Write(0:w463, 1:T14 {"Calibrated?"=FALSE, "IMU Detected?"=TRUE} ("element")) -> ()  [unwired: 3 in, 4 out]
            n155 = RT FIFO Write(0:w459, 1:T16 {"Command"=enum."Recalibrate", "Data"=0} ("element")) -> ()  [unwired: 3 in, 4 out]
          }
          frame "Configure Cal" {
            n156 = Bundle By Name(cluster=w469, "ADIS16448DevRef.Calibration Time"=w466) -> (w468:T13)
          }
        }
      }
    }
  }
  n157 = while {
    tunnel: w8 -> [w472]
    tunnel: [w471] -> w2
    stop <- w471 stop-if-true
    # "stop this VI when the VI calling StartComm goes idle"
    n158 = property class="VI"(reference=w472) -> ("Exec.State"=w474:T21)  [unwired: 1 in, 2 out]
    n159 = Wait (ms)(milliseconds to wait=u32 250) -> ()  [unwired: 1 out]
    n160 = Equal?(x=w474, y=T21."Idle" ("Execution:State")) -> (x = y?=w471:bool)
  }
  n161 = flat-sequence {
    tunnel: w2 -> [_]
    frame #0 {
      n162 = call <vilib>:"WPI_DigitalOutputRefNum Registry Get.vi"("refnum name"="448 Status LED") -> ("error out"=w481:errorcluster, "DigitalOutputDevRef"=w480:T17)  [unwired: 9 in]
      n163 = call <vilib>:"WPI_DigitalOutputClose.vi"("error in (no error)"=w481, "DigitalOutputDevRef"=w480) -> ("error out"=w476:errorcluster)  [unwired: 9 in]
      n164 = call <vilib>:"WPI_SPIRefNum Registry Get.vi"("error in (no error)"=w476, "refnum name"="AutoSPI") -> ("error out"=w478:errorcluster, "SPIDevRef"=w477:T12)  [unwired: 8 in]
      n165 = call <vilib>:"WPI_SPIClose.vi"("error in (no error)"=w478, "SPIDevRef"=w477) -> ()  [unwired: 9 in, 1 out]
    }
    frame #1 {
      n166 = Stop() -> ()  [unwired: 1 in]
    }
  }
